vi "Configure Stepped TimerDRV.vi"(8 "error in (no error)":errorcluster, 11 "TimerDRV in":refnum<class "TimerDRV.lvclass">) -> (0 "error out":errorcluster, 3 "TimerDRV out":refnum<class "TimerDRV.lvclass">)   [LabVIEW 2019, in "TimingDRV Engine.lvlib" / "TimerDRV.lvclass"]
uses:
  TimerDRV.lvclass
  TimerDRV.lvclass/TimerDRV.ctl
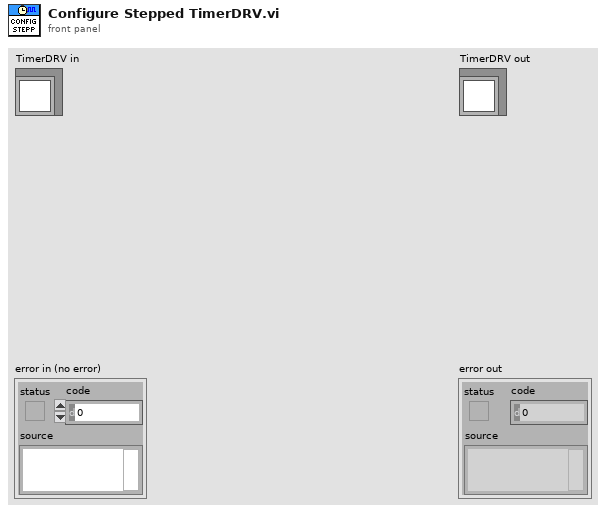
[diagram p1: front panel]
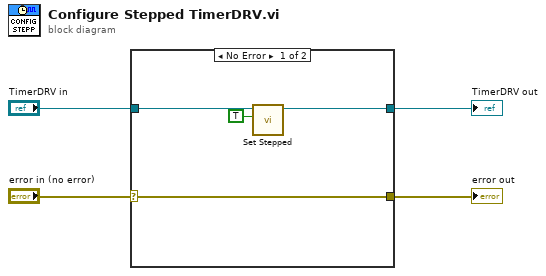
[diagram p0: block diagram]
diagram:
  n1 = case shown="No Error" "error in (no error)" {
    selector: "error in (no error)" -> [w8 w10]
    tunnel: [w8 w10] -> w3
    tunnel: [w6 w9] -> w1
    tunnel: "TimerDRV in" -> [w7 w9]
    frame No Error {
      n2 = call "Set Stepped.vi"("Stepped"=TRUE, "TimerDRV in"=w7) -> ("TimerDRV out"=w6:refnum<class "TimerDRV.lvclass">)  [unwired: 9 in]
    }
    frame Error {
    }
  }
  "error out" <- w3
  "TimerDRV out" <- w1
